vi "begin5PreparePassGamePlay.vi"(8 "error in (no error)":errorcluster, 9 "last command_interpreted":T1, 10 "Game":refnum<class "Game.lvclass">, 11 "5PreparePassGamePlay in":refnum<class "5PreparePassGamePlay.lvclass">) -> (0 "error out":errorcluster, 1 "BeginPreparePass?":bool, 2 "Game out":refnum<class "Game.lvclass">, 3 "5PreparePassGamePlay out":refnum<class "5PreparePassGamePlay.lvclass">)   [LabVIEW 2023, in "5PreparePassGamePlay.lvclass"]
uses:
  5PreparePassGamePlay.lvclass
  C:/Users/ebert/Documents/codes/SSL/repo/SSL_AI/Play_class/Play.lvclass
  Game_class/Game.lvclass
  Referee_class/command_interpreted.ctl
  Events_class/Possession.ctl
  Zone_class/zones.ctl
  Team_class/OffensivePlay.ctl
  Game_class/Game.lvclass/Game.ctl
  Referee_class/Referee.lvclass/Referee.ctl
  Parameters_class/Parameters.lvclass/Parameters.ctl
  Object_class/Object.lvclass/Object.ctl
  Team_class/Team.lvclass/Team.ctl
  Game_class/Read Referee.vi
  Game_class/Read Parameters.lvclass.vi
  Game_class/Read BallRef.vi
  Game_class/Read Utilities.lvclass.vi
  Game_class/Read OffensiveTeam.vi
  Game_class/Read EventsRef.vi
  Team_class/Read Evaluators.vi
  Team_class/Read RobotRef.vi
  Team_class/Read OffensivePlay.vi
  Team_class/Read currentBallZone.vi
  Object_class/Read position(x,y).vi
  Parameters_class/Read RollToPass.vi
  Referee_class/Read command_interpreted.vi
  Ally_class/Ally.lvclass
  C:/Users/ebert/Documents/codes/SSL/repo/SSL_AI/Team_class/Team.lvclass
  Ball_class/Ball.lvclass
  C:/Users/ebert/Documents/codes/SSL/repo/SSL_AI/Object_class/Object.lvclass
  Referee_class/Referee.lvclass
  Parameters_class/Parameters.lvclass
  Utilities_class/Utilities.lvclass
  Events_class/Events.lvclass
  NewSTP/Evaluators/Evaluator_class/Evaluator.lvclass
  Robot_class/Robot.lvclass
  Play_class/Play.lvclass
  Zone_class/Zone.lvclass
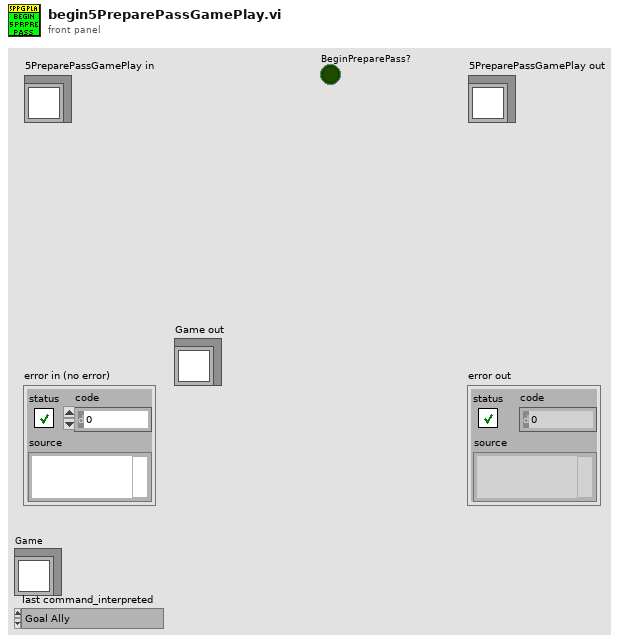
[diagram p1: front panel]
types:
  T1 = typedef "command_interpreted.ctl" = enum16{"Goal Ally", "Goal Enemy", "Ball Placement Enemy", "Ball Placement Ally", "Normal Half Time", "Extra Time  Break", "Extra Half Time", "None", "Post Game", "PKA Normal Start", "Prepare Kickoff Ally", "PKE Normal Start", "Prepare Kickoff Enemy", "Force Start", "Halt", "Timeout", "Prepare Penalty Ally", "Prepare Penalty Enemy", "PPA NormalStart", "PPE Normal Start", "Indirect Free Ally", "Direct Free Enemy", "Direct Free Ally", "Indirect Free Enemy", "Stop"}
  T2 = typedef "OffensivePlay.ctl" = enum16{"5RobotsPassGamePlay", "5PreparePassGame", "5RobotsKeeperGame", "KeeperPassToStriker", "5RobotsNormalGamePlay", "PrepareKeeperPass", "ACBPass", "ABCPass", "PrepareTriplePass", "TableWithStriker", "TableWith2ndStrikerPlay", "PrepareDoublePass", "PrepareRollToPass", "SimplePass", "PreparePass", "PassToStriker", "BallOutOfField", "PassTo2ndStriker", "StopOffensive", "Prepare Penalty Enemy", "EnemyPossessionAtEnemyField", "EnemyPossesionAtOurField", "TestPlay", "PreparePenaltyAlly", "KickPenaltyAlly", "PrepareKickoffAlly", "PrepareKickoffEnemy", "IndirectEnemy", "DirectEnemy", "PreparePassInGame1", "NormalGame", "DirectKick", "Pass", "Halt", "Timeout", "PassPlay", "PenaltyEnemy"}
  T3 = typedef "Zone.lvclass/zones.ctl" = enum16{"leftMidField", "rightMidField", "MidField", "leftWing", "rightWing", "LeftSide", "RightSide", "Field", "Size"}
  T4 = typedef "Events.lvclass/Possession.ctl" = enum16{"OurPossession", "TheirPossession", "Contended", "Loose"}
  T5 = typedef "STPParameters.ctl" = cluster{"Skills":T6, "TestSkill":T8, "Events":cluster{"distanceToBallPossession":dbl, "timeForPossessionThreshold":dbl}, "Criteria":cluster{"OpenAngleToGoal":cluster{"minAngle":dbl, "maxAngle":dbl, "minEvaluation":dbl}, "PassDistance":cluster{"maxDistance":dbl, "minDistance":dbl}, "ShotInterception":cluster{"shotSpeed":dbl, "minEnemySpeed":dbl, "minEvaluation":dbl, "maxEnemySpeed":dbl}, "OneTouchShot":cluster{"MaxAngle":dbl, "minEvaluation":dbl}, "PassInterception":cluster{"minEnemySpeed":dbl, "maxEnemySpeed":dbl, "chipPassDistance":dbl, "chipPassEval":dbl, "minEvaluation":dbl}}, "minPassSpeed":dbl, "maxPassSpeed":dbl, "AllyTeamIds":T9[], "ReceiverSpeed":dbl, "minEvaluationToShoot":dbl, "maxDefendersNumber":u8}
  T6 = typedef "Skills.ctl" = cluster{"CirculateBall":T7, "ProtectBall":cluster{"DistanceFromBall":dbl}}
  T7 = typedef "CIrculateSkillParameters.ctl" = cluster{"rotationAngle":dbl, "velocityFactor":dbl, "OrientationFactor":dbl}
  T8 = typedef "TestSkills.ctl" = enum16{"AlignSkill", "PassSkill", "CirculateBall", "OneTouchShotSkill", "KickToSkill_v2", "ShootSkill", "InterceptBall", "Exit", "GoToSkill_v2"}
  T9 = typedef "AllyTeam.ctl" = enum16{"Keeper", "Defender", "Attacker"}
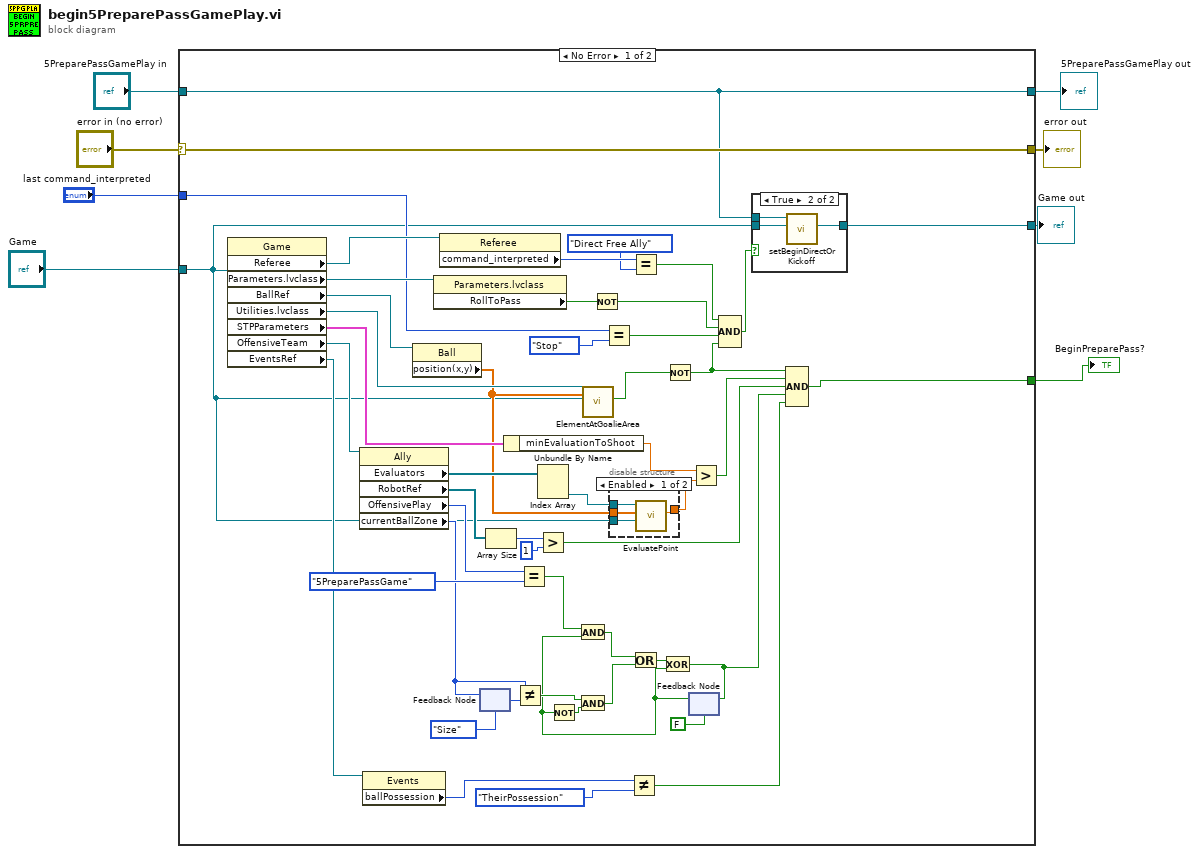
[diagram p0: block diagram]
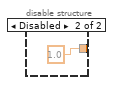
[diagram p2: hidden frame]
diagram:
  n1 = case shown="No Error" "error in (no error)" {
    selector: "error in (no error)" -> [w58 w69]
    tunnel: [w58 w69] -> w7
    tunnel: [w52 w68] -> w5
    tunnel: "5PreparePassGamePlay in" -> [w52 w68]
    tunnel: "Game" -> [w9 _]
    tunnel: "last command_interpreted" -> [w53 _]
    tunnel: [w51 _] -> w3
    tunnel: [w25 _] -> w1
    frame No Error {
      n2 = property class="Game"(reference=w9) -> ("Referee"=w57:refnum<class "Referee.lvclass">, "Parameters.lvclass"=w55:refnum<class "Parameters.lvclass">, "BallRef"=w50:refnum<class "Ball.lvclass">, "Utilities.lvclass"=w48:refnum<class "Utilities.lvclass">, "STPParameters"=w39:T5, "OffensiveTeam"=w40:refnum<class "Ally.lvclass">, "EventsRef"=w33:refnum<class "Events.lvclass">)  [unwired: 1 in, 2 out]
      n3 = property class="Ally"(reference=w40) -> ("Evaluators"=w42:refnum<class "Evaluator.lvclass">[], "RobotRef"=w30:refnum<class "Robot.lvclass">[], "OffensivePlay"=w15:T2, "currentBallZone"=w14:T3)  [unwired: 1 in, 2 out]
      n4 = property class="Events"(reference=w33) -> ("ballPossession"=w32:T4)  [unwired: 1 in, 2 out]
      n5 = property class="Ball"(reference=w50) -> ("position(x,y)"=w38:dbl[])  [unwired: 1 in, 2 out]
      n6 = property class="Parameters.lvclass"(reference=w55) -> ("RollToPass"=w54:bool)  [unwired: 1 in, 2 out]
      n7 = property class="Referee"(reference=w57) -> ("command_interpreted"=w47:T1)  [unwired: 1 in, 2 out]
      n8 = feedback-in #1(w14) -> ()
      n9 = feedback #1(zones."Size" ("currentBallZone")) -> (w23:T3)
      n10 = Array Size(array=w30) -> (size(s)=w29:i32)
      n11 = Unbundle By Name(w39) -> ("minEvaluationToShoot"=w37:dbl)
      n12 = Not Equal?(x=w14, y=w23) -> (x != y?=w17:bool)
      n13 = Equal?(x=w15, y=OffensivePlay."5PreparePassGame") -> (x = y?=w10:bool)
      n14 = Index Array(array=w42) -> (element #2=w41:refnum<class "Evaluator.lvclass">)  [unwired: 2 in, 1 out]
      n15 = Greater?(x=w29, y=1) -> (0:w27:bool)
      n16 = call "ElementAtGoalieArea.vi"("Elemento pos."=w38, "Game"=w9, "Utilities in"=w48) -> ("Element at any goalkeeper area ?"=w49:bool)  [unwired: 4 in, 4 out]
      n17 = Not(x=w54) -> (.not. x?=w44:bool)
      n18 = Equal?(x=w53, y=command_interpreted."Stop" ("command_interpreted")) -> (x = y?=w43:bool)
      n19 = disable-structure shown="Enabled" {
        disable-tunnel: w41 -> [w62 _]
        disable-tunnel: w9 -> [w61 _]
        disable-tunnel: w38 -> [w60 _]
        disable-tunnel: [w59 1.0 ("Evaluation")] -> w36
        frame Enabled {
          n20 = call-dynamic "EvaluatePoint.vi"("Game"=w61, "Point"=w60, "Evaluator in"=w62) -> ("Evaluation"=w59:dbl)  [unwired: 6 in, 2 out]
        }
        frame Disabled {
        }
      }
      n21 = Not Equal?(x=w32, y=Possession."TheirPossession") -> (x != y?=w26:bool)
      n22 = Equal?(x=w47, y=command_interpreted."Direct Free Ally") -> (x = y?=w46:bool)
      n23 = Not(x=w49) -> (.not. x?=w35:bool)
      n24 = feedback #2(FALSE) -> (w11:bool)
      n25 = Not(x=w11) -> (.not. x?=w13:bool)
      n26 = And(x=w10, y=w11) -> (x .and. y?=w12:bool)
      n27 = And(x=w17, y=w13) -> (x .and. y?=w16:bool)
      n28 = Or(x=w12, y=w16) -> (x .or. y?=w19:bool)
      n29 = Exclusive Or(1:w11, 2:w19) -> (0:w20:bool)
      n30 = feedback-in #2(w20) -> ()
      n31 = Greater?(x=w37, y=w36) -> (0:w34:bool)
      n32 = Compound Arithmetic op=AND(w46, w44, w43, w35) -> (w24:bool)
      n33 = case shown="True" w24 {
        tunnel: w52 -> [_ w67]
        tunnel: w9 -> [w64 w66]
        tunnel: [w64 w65] -> w51
        frame False {
        }
        frame True {
          n34 = call "setBeginDirectOrKickoff.vi"("Game in"=w66, "Play in"=w67) -> ("Game out"=w65:refnum<class "Game.lvclass">)  [unwired: 7 in, 2 out]
        }
      }
      n35 = Compound Arithmetic op=AND(w35, w34, w27, w20, w26) -> (w25:bool)
    }
    frame Error {
    }
  }
  "error out" <- w7
  "5PreparePassGamePlay out" <- w5
  "BeginPreparePass?" <- w1
  "Game out" <- w3
